vi "Measurement-TE.vi"(3 "Ctl Refnum":refnum<vi>, 5 "升温速率":dbl=80.0, 6 "Boolean":bool, 7 "目标温度":dbl=80.0, 8 "error in (no error)":errorcluster caption="错误输入（无错误）", 9 "高温 2":refnum<visa-resource-name> caption="高温地址2", 10 "高温":refnum<visa-resource-name> caption="高温地址1", 11 "低温地址":refnum<visa-resource-name>="COM3") -> (0 "error out":errorcluster caption="错误输出")   [LabVIEW 2017]
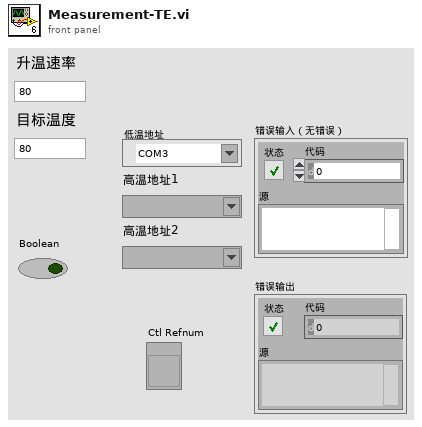
[diagram p1: front panel]
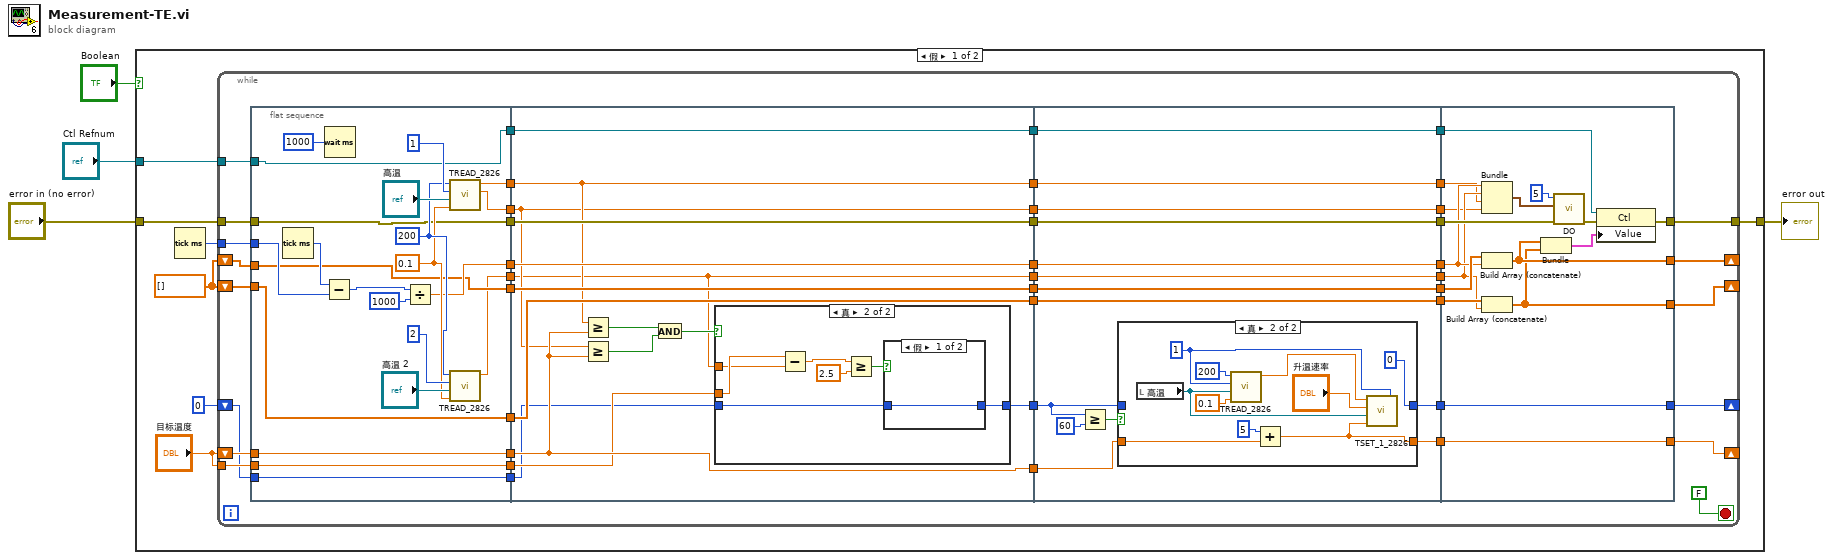
[diagram p0: block diagram]
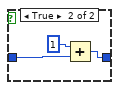
[diagram p3: hidden frame]
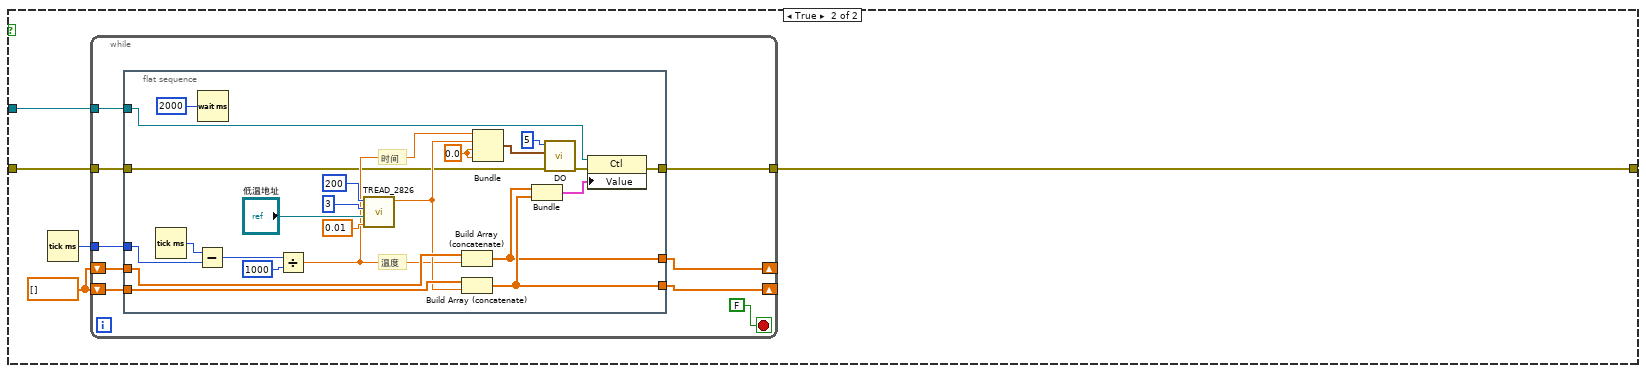
[diagram p5: hidden frame]
diagram:
  n1 = case shown="假" "Boolean" {
    tunnel: "Ctl Refnum" -> [w9 w153]
    tunnel: [w8 w149] -> w2
    tunnel: "error in (no error)" -> [w7 w150]
    frame False {
      w10 = dbl[] []
      n2 = Tick Count (ms)() -> (millisecond timer value=w11:u32)
      n3 = while {
        tunnel: w11 -> [w55]
        shift-right: [w54] -> _
        shift-left: w10 -> [w49]
        shift-right: [w53] -> _
        shift-left: w10 -> [w48]
        tunnel: w9 -> [w50]
        tunnel: [w52] -> w8
        tunnel: w7 -> [w47]
        shift-right: [w15] -> _
        shift-left: "目标温度" -> [w51]
        tunnel: "目标温度" -> [w36]
        shift-right: [w12] -> _
        shift-left: 0 -> [w35]
        stop <- FALSE stop-if-true
        n4 = flat-sequence {
          tunnel: w55 -> [w77]
          tunnel: [w67] -> w46
          tunnel: w51 -> [w67]
          tunnel: [w66] -> w45
          tunnel: w50 -> [w66]
          tunnel: [w65] -> w44
          tunnel: [w64] -> w43
          tunnel: w49 -> [w64]
          tunnel: [w63] -> w42
          tunnel: [w62] -> w41
          tunnel: w48 -> [w62]
          tunnel: [w61] -> w40
          tunnel: w47 -> [w61]
          tunnel: [w60] -> w39
          tunnel: [w59] -> w38
          tunnel: [w58] -> w37
          tunnel: w36 -> [w58]
          tunnel: w35 -> [w57]
          tunnel: [w57] -> w34
          tunnel: w46 -> [w88]
          tunnel: [w88] -> w33
          tunnel: w45 -> [w93]
          tunnel: [w93] -> w32
          tunnel: w44 -> [w92]
          tunnel: [w92] -> w30
          tunnel: w43 -> [w91]
          tunnel: [w91] -> w28
          tunnel: w42 -> [w82]
          tunnel: [w82] -> w26
          tunnel: w41 -> [w90]
          tunnel: [w90] -> w24
          tunnel: w40 -> [w89]
          tunnel: [w89] -> w22
          tunnel: w39 -> [w87]
          tunnel: [w87] -> w20
          tunnel: w38 -> [w86]
          tunnel: [w86] -> w18
          tunnel: w37 -> [w81]
          tunnel: w34 -> [w80]
          tunnel: [w79] -> w16
          tunnel: w33 -> [w108]
          tunnel: w32 -> [w119]
          tunnel: [w119] -> w31
          tunnel: w30 -> [w118]
          tunnel: [w118] -> w29
          tunnel: w28 -> [w117]
          tunnel: [w117] -> w27
          tunnel: w26 -> [w116]
          tunnel: [w116] -> w25
          tunnel: w24 -> [w115]
          tunnel: [w115] -> w23
          tunnel: w22 -> [w114]
          tunnel: [w114] -> w21
          tunnel: w20 -> [w113]
          tunnel: [w113] -> w19
          tunnel: w18 -> [w112]
          tunnel: [w112] -> w17
          tunnel: w16 -> [w109]
          tunnel: [w107] -> w14
          tunnel: [w106] -> w13
          tunnel: [w145] -> w54
          tunnel: [w143] -> w53
          tunnel: [w148] -> w52
          tunnel: w31 -> [w147]
          tunnel: w29 -> [w138]
          tunnel: w27 -> [w144]
          tunnel: w25 -> [w137]
          tunnel: w23 -> [w142]
          tunnel: w21 -> [w140]
          tunnel: w19 -> [w136]
          tunnel: w17 -> [w135]
          tunnel: [w133] -> w15
          tunnel: w14 -> [w133]
          tunnel: w13 -> [w132]
          tunnel: [w132] -> w12
          frame #0 {
            w68 = 0.1
            w69 = 200
            n5 = Tick Count (ms)() -> (millisecond timer value=w78:u32)
            n6 = Subtract(x=w78, y=w77) -> (x-y=w76:u32)
            n7 = Wait (ms)(milliseconds to wait=u32 1000 ("等待时间（毫秒）")) -> ()  [unwired: 1 out]
            n8 = Divide(x=w76, y=u32 1000) -> (x/y=w65:dbl)
            n9 = call "TREAD_2826.vi"("Unknown Param 2"=w68, "VISA resource name"="高温", "Address No."=i8 1, "Unknown Param"=w69) -> ("SV"=w59:dbl, "PV"=w60:dbl)  [unwired: 2 out]
            n10 = call "TREAD_2826.vi"("Unknown Param 2"=w68, "VISA resource name"="高温 2", "Address No."=i8 2, "Unknown Param"=w69) -> ("PV"=w63:dbl)  [unwired: 3 out]
          }
          frame #1 {
            n11 = Greater Or Equal?(x=w87, y=w88) -> (x >= y?=w85:bool)
            n12 = Greater Or Equal?(x=w86, y=w88) -> (x >= y?=w84:bool)
            n13 = And(x=w85, y=w84) -> (x .and. y?=w83:bool)
            n14 = case shown="真" w83 {
              tunnel: w82 -> [_ w100]
              tunnel: w81 -> [_ w101]
              tunnel: w80 -> [w94 w96]
              tunnel: [w94 w95] -> w79
              frame False {
              }
              frame True {
                n15 = Subtract(x=w101, y=w100) -> (x-y=w99:dbl)
                n16 = Greater Or Equal?(x=w99, y=2.5) -> (x >= y?=w97:bool)
                n17 = case shown="假" w97 {
                  tunnel: w96 -> [w102 w104]
                  tunnel: [w102 w103] -> w95
                  frame False {
                  }
                  frame True {
                    n18 = Add(x=1, y=w104) -> (x+y=w103:i32)
                  }
                }
              }
            }
          }
          frame #2 {
            n19 = Greater Or Equal?(x=w109, y=60) -> (x >= y?=w110:bool)
            n20 = case shown="真" w110 {
              tunnel: w109 -> [w121 _]
              tunnel: [w121 0] -> w106
              tunnel: w108 -> [w120 w124]
              tunnel: [w120 w123] -> w107
              frame False {
              }
              frame True {
                w127 = i8 1 ("Address No.")
                n21 = local read "高温"() -> (w122:refnum<visa-resource-name>)
                n22 = call "TREAD_2826.vi"("Unknown Param 2"=0.1, "VISA resource name"=w122, "Address No."=w127, "Unknown Param"=200) -> ("PV"=w128:dbl)  [unwired: 3 out]
                n23 = Add(x=5, y=w124) -> (x+y=w123:dbl)
                n24 = call "TSET_1_2826.vi"("Address No."=w127, "T-Ending, C"=w123, "VISA resource name"=w122, "cooling/heating rate, C/min"="升温速率", "T-Starting, C"=w128) -> ()
              }
            }
          }
          frame #3 {
            n25 = Bundle(w138, "PV"=w137, "PV"=w136, "SV"=w135) -> (w134:cluster{dbl, "PV":dbl, "PV":dbl, "SV":dbl})  [unwired: 1 in]
            n26 = Build Array (concatenate)(w144, w138) -> (w145:dbl[])
            n27 = Build Array (concatenate)(w142, w137) -> (w143:dbl[])
            n28 = Bundle(w145, w143) -> (w146:cluster{dbl[], dbl[]})  [unwired: 1 in]
            n29 = call "DO.vi"("error in (no error)"=w140, "数据输出"=w134, "功能编号"=5) -> ("error out"=w141:errorcluster)  [unwired: 8 in]
            n30 = property class="Ctl"(reference=w147, error in=w141, "Value"=w146) -> (error out=w148:errorcluster)  [unwired: 1 out]
          }
        }
      }
    }
    frame True {
      w152 = dbl[] []
      n31 = Tick Count (ms)() -> (millisecond timer value=w151:u32)
      n32 = while {
        tunnel: w151 -> [w161]
        shift-right: [w158] -> _
        shift-left: w152 -> [w160]
        shift-right: [w157] -> _
        shift-left: w152 -> [w159]
        tunnel: w153 -> [w156]
        tunnel: w150 -> [w155]
        tunnel: [w154] -> w149
        stop <- FALSE stop-if-true
        n33 = flat-sequence {
          tunnel: w161 -> [w184]
          tunnel: w160 -> [w180]
          tunnel: w159 -> [w179]
          tunnel: w156 -> [w170]
          tunnel: [w177] -> w158
          tunnel: [w176] -> w157
          tunnel: w155 -> [w164]
          tunnel: [w163] -> w154
          frame #0 {
            w168 = 0.0
            # "时间"
            # "温度"
            n34 = Tick Count (ms)() -> (millisecond timer value=w185:u32)
            n35 = Subtract(x=w185, y=w184) -> (x-y=w183:u32)
            n36 = Wait (ms)(milliseconds to wait=u32 2000 ("等待时间（毫秒）")) -> ()  [unwired: 1 out]
            n37 = Divide(x=w183, y=u32 1000) -> (x/y=w171:dbl)
            n38 = call "TREAD_2826.vi"("Unknown Param 2"=0.01, "VISA resource name"="低温地址", "Address No."=i8 3, "Unknown Param"=200) -> ("PV"=w172:dbl)  [unwired: 3 out]
            n39 = Build Array (concatenate)(w179, w171) -> (w176:dbl[])
            n40 = Build Array (concatenate)(w180, w172) -> (w177:dbl[])
            n41 = Bundle(w171, "PV"=w172, w168, w168) -> (w166:cluster{dbl, "PV":dbl, dbl, dbl})  [unwired: 1 in]
            n42 = Bundle(w176, w177) -> (w169:cluster{dbl[], dbl[]})  [unwired: 1 in]
            n43 = call "DO.vi"("error in (no error)"=w164, "数据输出"=w166, "功能编号"=5) -> ("error out"=w165:errorcluster)  [unwired: 8 in]
            n44 = property class="Ctl"(reference=w170, error in=w165, "Value"=w169) -> (error out=w163:errorcluster)  [unwired: 1 out]
          }
        }
      }
    }
  }
  "error out" <- w2
